vi "Average Encoders.vi"() -> (1 "Counts":dbl, 2 "Period":dbl)   [LabVIEW 2013]
panel:
  in  "One Encoder Mode":bool=TRUE
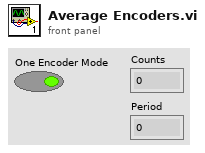
[diagram p1: front panel]
types:
  T1 = typedef "WPI_CounterDevRef.ctl" = cluster{"DevStatus":errorcluster, "CntIndex":T2}
  T2 = typedef "FPGA_CounterCtrSystemIndex.ctl" = enum8{"Ctr 0", "Ctr 1", "Ctr 2", "Ctr 3", "Ctr 4", "Ctr 5", "Ctr 6", "Ctr 7", "Invalid"}
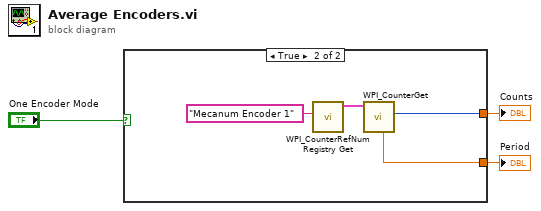
[diagram p0: block diagram]
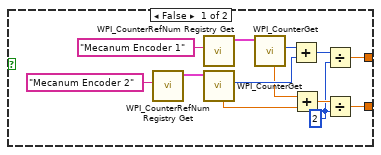
[diagram p2: hidden frame]
diagram:
  n1 = case shown="True" "One Encoder Mode" {
    tunnel: [w5 w18] -> w3
    tunnel: [w4 w17] -> w2
    frame False {
      w7 = 2
      n2 = call <vilib>:"WPI_CounterRefNum Registry Get.vi"("refnum name"="Mecanum Encoder 2") -> ("CounterDevRef"=w14:T1)  [unwired: 9 in, 1 out]
      n3 = call <vilib>:"WPI_CounterRefNum Registry Get.vi"("refnum name"="Mecanum Encoder 1") -> ("CounterDevRef"=w13:T1)  [unwired: 9 in, 1 out]
      n4 = call <vilib>:"WPI_CounterGet.vi"("CounterDevRef in"=w14) -> ("Value"=w11:i32, "Period (sec)"=w9:dbl)  [unwired: 5 in, 4 out]
      n5 = call <vilib>:"WPI_CounterGet.vi"("CounterDevRef in"=w13) -> ("Value"=w12:i32, "Period (sec)"=w10:dbl)  [unwired: 5 in, 4 out]
      n6 = Add(x=w12, y=w11) -> (x+y=w6:i32)
      n7 = Add(x=w10, y=w9) -> (x+y=w8:dbl)
      n8 = Divide(x=w6, y=w7) -> (x/y=w5:dbl)
      n9 = Divide(x=w8, y=w7) -> (x/y=w4:dbl)
    }
    frame True {
      n10 = call <vilib>:"WPI_CounterRefNum Registry Get.vi"("refnum name"="Mecanum Encoder 1") -> ("CounterDevRef"=w19:T1)  [unwired: 9 in, 1 out]
      n11 = call <vilib>:"WPI_CounterGet.vi"("CounterDevRef in"=w19) -> ("Value"=w18:i32, "Period (sec)"=w17:dbl)  [unwired: 5 in, 4 out]
    }
  }
  "Counts" <- w3
  "Period" <- w2
